vi "Notifier to Command String.vi"(10 "Control by hand?":bool, 11 "NotifierReff":T2) -> (3 "String":string)   [LabVIEW 2013]
doc: "Takes the MB sail and rudder commands (-1 to 1 for rudder, 0 to 1 for sails) and translates that into a command string for the arbotix board.\n\nEric Schneider, April 2014"
uses:
  Data/TypeDefs/Notifiers.ctl
  Data/TypeDefs/UTM Location.ctl
  Data/TypeDefs/Sail Set Suggestions.ctl
  Data/TypeDefs/Rudder Set Suggestions.ctl
  Data/TypeDefs/OverrideInformation.ctl
  Data/TypeDefs/OverrideMode.ctl
  Data/TypeDefs/MotorSetup.ctl
  Data/TypeDefs/DynamixelSetupInfo.ctl
  Data/TypeDefs/AirmarStatus.ctl
panel:
  in  "Suggested Rudder Setpoint":T1 min=-1.0 max=1.0 scale=1.0..-1.0
  in  "MainSailSuggestion":dbl
  in  "JibSailSuggestion":dbl
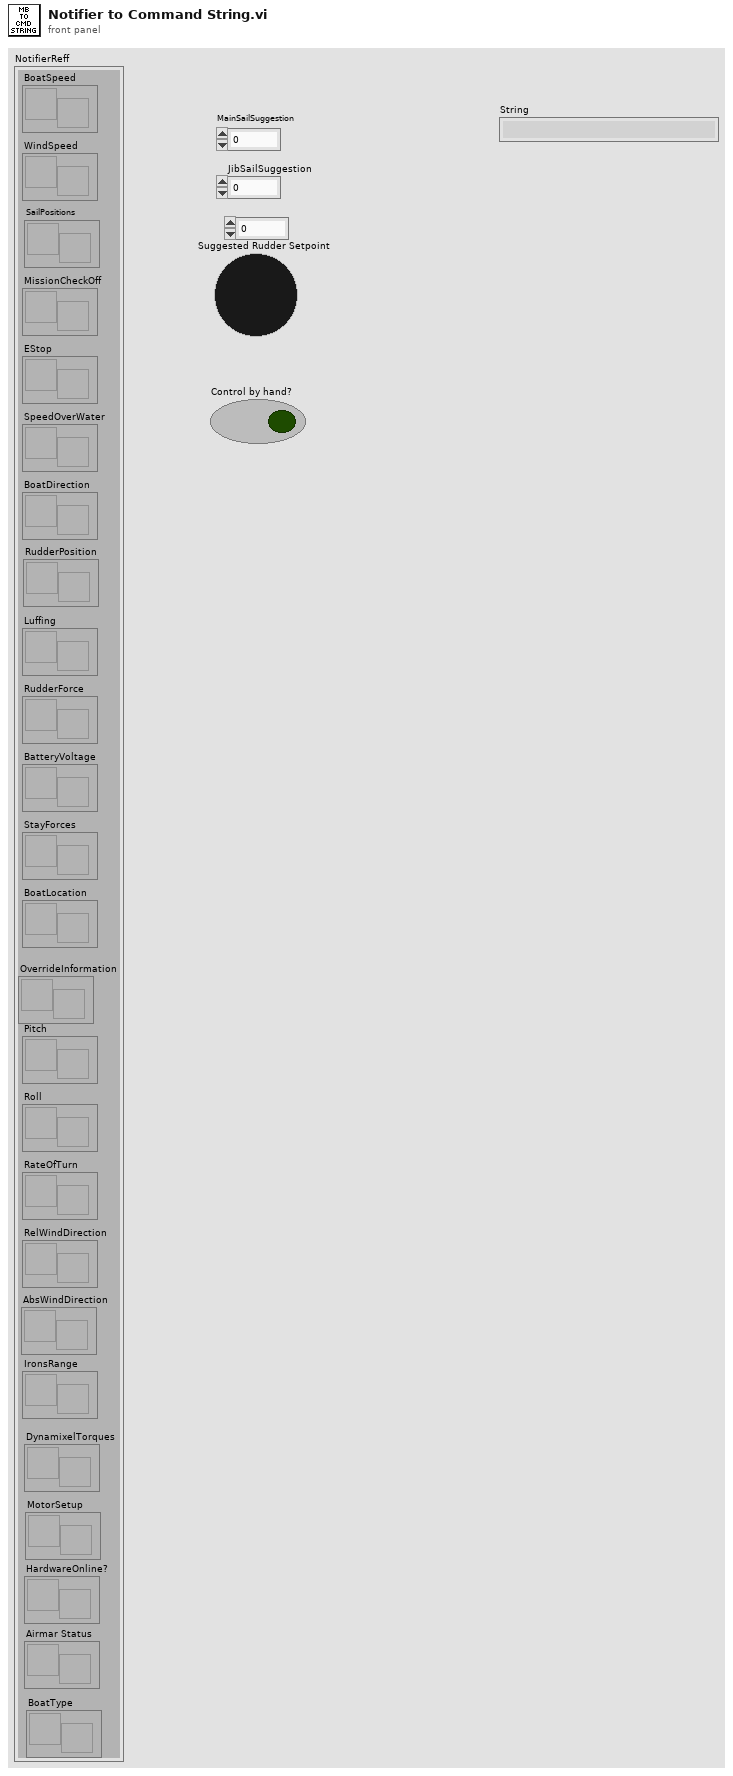
[diagram p1: front panel]
types:
  T1 = typedef "Rudder Set Suggestions.ctl" = dbl
  T2 = typedef "Notifiers.ctl" = cluster{"BoatSpeed":refnum<notifier>, "WindSpeed":refnum<notifier>, "MissionCheckOff":refnum<notifier>, "EStop":refnum<notifier>, "SpeedOverWater":refnum<notifier>, "BoatDirection":refnum<notifier>, "Luffing":refnum<notifier>, "RudderForce":refnum<notifier>, "BatteryVoltage":refnum<notifier>, "StayForces":refnum<notifier>, "BoatLocation":refnum<notifier>, "Pitch":refnum<notifier>, "Roll":refnum<notifier>, "RateOfTurn":refnum<notifier>, "RelWindDirection":refnum<notifier>, "SailPositions":refnum<notifier>, "RudderPosition":refnum<notifier>, "IronsRange":refnum<notifier>, "AbsWindDirection":refnum<notifier>, "OverrideInformation":refnum<notifier>, "DynamixelTorques":refnum<notifier>, "HardwareOnline?":refnum<notifier>, "MotorSetup":refnum<notifier>, "Airmar Status":refnum<notifier>, "BoatType":refnum<notifier>}
  T3 = typedef "Sail Set Suggestions.ctl" = cluster{"MainSailSuggestion":dbl, "JibSailSuggestion":dbl}
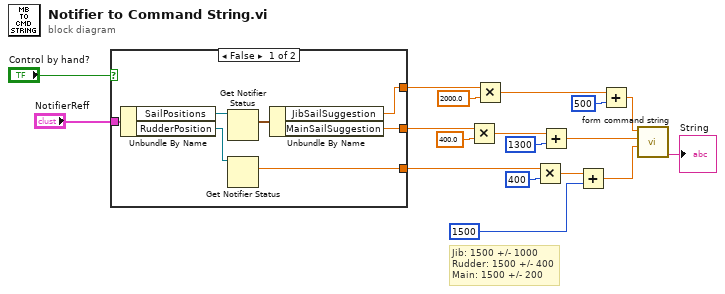
[diagram p0: block diagram]
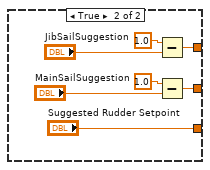
[diagram p2: hidden frame]
diagram:
  # "Jib: 1500 +/- 1000\nRudder: 1500 +/- 400\nMain: 1500 +/- 200"
  n1 = case shown="False" "Control by hand?" {
    tunnel: "NotifierReff" -> [w23 _]
    tunnel: [w21 "Suggested Rudder Setpoint"] -> w15
    tunnel: [w20 w26] -> w9
    tunnel: [w19 w29] -> w2
    frame False {
      n2 = Unbundle By Name(w23) -> ("SailPositions"=w25:refnum<notifier>, "RudderPosition"=w24:refnum<notifier>)
      n3 = Get Notifier Status(notifier=w25) -> (current notification=w22:T3)  [unwired: 1 in, 4 out]
      n4 = Get Notifier Status(notifier=w24) -> (current notification=w21:T1)  [unwired: 1 in, 4 out]
      n5 = Unbundle By Name(w22) -> ("JibSailSuggestion"=w20:dbl, "MainSailSuggestion"=w19:dbl)
    }
    frame True {
      n6 = Subtract(x=1.0, y="JibSailSuggestion") -> (x-y=w26:dbl)
      n7 = Subtract(x=1.0, y="MainSailSuggestion") -> (x-y=w29:dbl)
    }
  }
  n8 = Multiply(x=w2, y=400.0) -> (x*y=w4:dbl)
  n9 = Multiply(x=w9, y=2000.0) -> (x*y=w8:dbl)
  n10 = Multiply(x=w15, y=400) -> (x*y=w13:T1)
  n11 = Add(x=w4, y=1300) -> (x+y=w3:dbl)
  n12 = Add(x=w13, y=1500) -> (x+y=w12:T1)
  n13 = Add(x=w8, y=500) -> (x+y=w7:dbl)
  n14 = call "form command string.vi"("Rudder"=w12, "Main sheet"=w3, "Jib Sheet"=w7) -> ("String"=→"String":string)  [unwired: 5 in, 3 out]
